vi "GA Arc XYC.vi"(0 "nCrdNum":i16, 1 "yCenter":dbl, 2 "synVel":dbl, 3 "velEnd":dbl, 5 "x":i32, 7 "y":i32, 9 "xCenter":dbl, 10 "segNum":i32, 11 "error in (no error)":errorcluster caption="错误输入（无错误）", 12 "circleDir":i16, 13 "synAcc":dbl, 14 "FifoIndex":i16) -> (4 "function return":i32, 15 "error out":errorcluster caption="错误输出")   [LabVIEW 2015, in "GAS.lvlib"]
doc: "extern \"C\" __declspec(dllimport) int GA_ArcXYC(short nCrdNum,long x,long y,double xCenter,double yCenter,short circleDir,double synVel,double synAcc,double velEnd=0,short FifoIndex=0,long segNum = 0);"
uses:
  <userlib>/BP_GAS/GAS.lvlib
  <userlib>/BP_GAS/GAS.dll
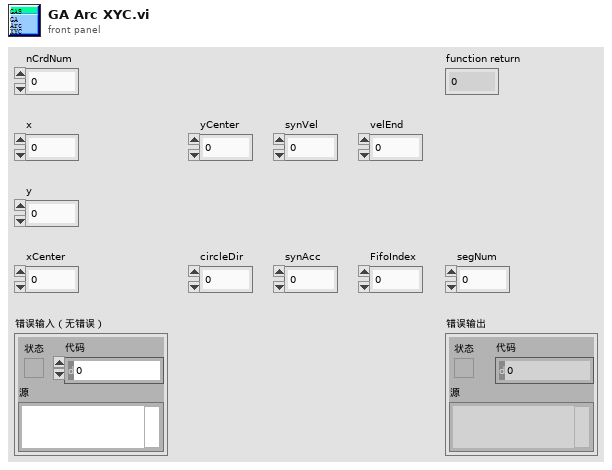
[diagram p1: front panel]
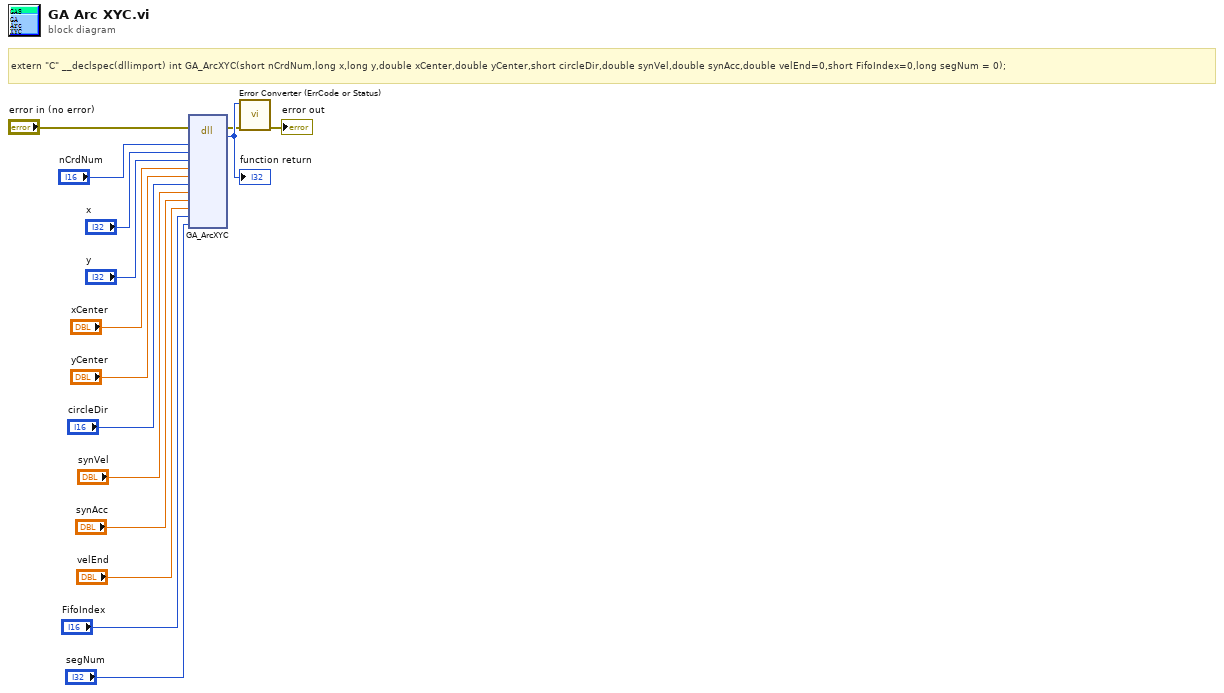
[diagram p0: block diagram]
diagram:
  # "extern \"C\" __declspec(dllimport) int GA_ArcXYC(short nCrdNum,long x,long y,double xCenter,double yCenter,short circleDir,double synVel,double synAcc,double velEnd=0,short FifoIndex=0,long segNum = 0);"
  n1 = dll-call lib="E:/Program Files (x86)/National Instruments/LabVIEW 2015/user.lib/BP_GAS/GAS.*" fn="GA_ArcXYC"(error in="error in (no error)", "nCrdNum"="nCrdNum", "x"="x", "y"="y", "xCenter"="xCenter", "yCenter"="yCenter", "circleDir"="circleDir", "synVel"="synVel", "synAcc"="synAcc", "velEnd"="velEnd", "FifoIndex"="FifoIndex", "segNum"="segNum") -> (error out=w2:errorcluster, w15:i32)  [unwired: 13 in, 1 out]
  "function return" <- w15
  n2 = call "Error Converter (ErrCode or Status).vi"("error in (no error)"=w2, "error code"=w15) -> ("error out"=→"error out":errorcluster)  [unwired: 9 in]
